vi "TCP Read - Specified Number of Bytes.vi"(8 "error in":errorcluster, 9 "Timeout ms (default 50ms)":i32=50, 10 "Bytes to Read":i32, 11 "TCP Network Connection in":refnum<k5>) -> (0 "error out":errorcluster, 2 "Unsigned Byte Array":u8[](array[numeric]), 3 "TCP Network Connection out":refnum<k5>)   [LabVIEW 2017, in "Communications Library.lvlib"]
doc: "Reads a specified number of bytes from the port. \n\nIf a smaller number of bytes are received, timeout will be true and a partial data set will be returned."
uses:
  Communications Library.lvlib
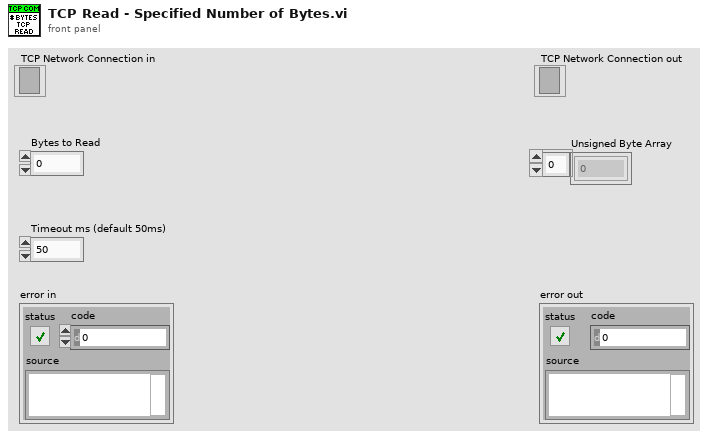
[diagram p1: front panel]
types:
  T1 = enum16{"Standard", "Buffered", "CRLF", "Immediate"}
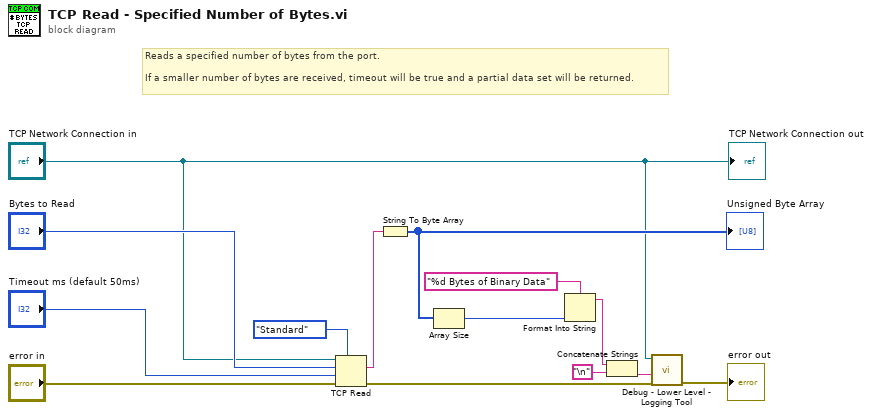
[diagram p0: block diagram]
diagram:
  # "Reads a specified number of bytes from the port. \n\nIf a smaller number of bytes are received, timeout will be true and a partial data set will be returned."
  n1 = TCP Read(connection ID="TCP Network Connection in", bytes to read="Bytes to Read", error in (no error)="error in", 7:T1."Standard" ("mode (standard)"), 9:"Timeout ms (default 50ms)") -> (data out=w12:string, error out=w9:errorcluster)  [unwired: 1 out]
  n2 = String To Byte Array(string=w12) -> (unsigned byte array=w7:u8[])
  "Unsigned Byte Array" <- w7
  n3 = Array Size(array=w7) -> (size(s)=w6:i32)
  n4 = Format Into String(format string="%d Bytes of Binary Data", w6) -> (resulting string=w2:string)  [unwired: 2 in, 1 out]
  n5 = Concatenate Strings(w2, "\n") -> (w3:string)
  n6 = call "Debug - Lower Level - Logging Tool.vi"("Error In"=w9, "Data Received"=w3, "TCP Network Connecion In"="TCP Network Connection in") -> ("Error Out"=→"error out":errorcluster)  [unwired: 7 in, 1 out]
  "TCP Network Connection out" <- "TCP Network Connection in"
